vi "SFOAE-Init Level.vi"(0 "AO Runtime in":T2, 7 "DataProc In":T1, 11 "error in (no error)":errorcluster, 12 "Seq Step":i32, 13 "Lp (dB SPL)":cluster{"Min":dbl, "Max":dbl, "Step":dbl}) -> (3 "Lp":dbl, 4 "AO Runtime out":T2, 8 "Continue?":bool, 14 "DataProc Out":T1, 15 "error out":errorcluster)   [LabVIEW 2020]
uses:
  Typedefs/SFOAE-AO Runtime Data.ctl
  Typedefs/SFOAE-Data Processing.ctl
  epl-vi-lib/PXI DAQ VIs/DAQ Engine VIs/PXI Globals.vi
  epl-vi-lib/Utility VIs/Math VIs/dB to Linear (scalar).vi
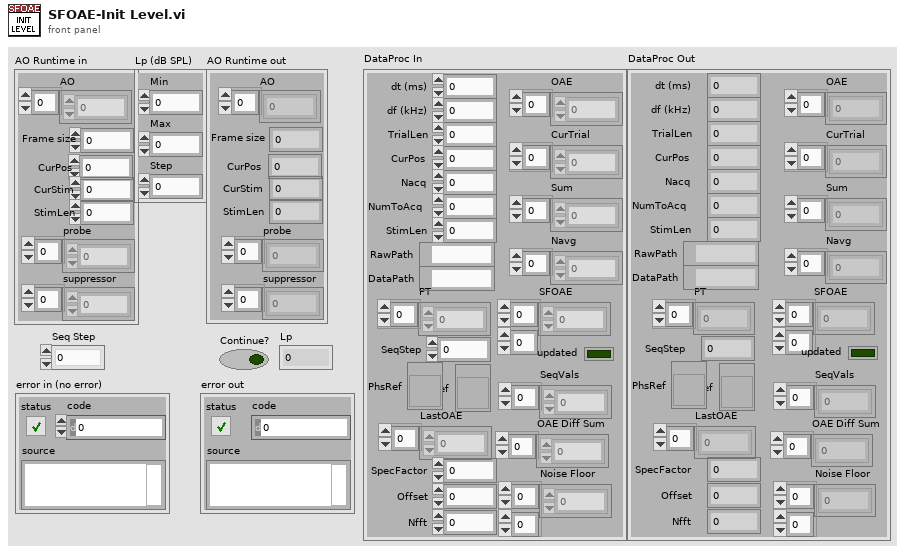
[diagram p1: front panel]
types:
  T1 = typedef "SFOAE-Data Processing.ctl" = cluster{"dt (ms)":dbl, "TrialLen":i32, "PT":cdb[], "CurPos":i32, "Sum":dbl[], "Navg":dbl[], "Nacq":i32, "RawPath":path, "DataPath":path, "NumToAcq":i32, "OAE":dbl[], "CurTrial":dbl[], "StimLen":i32, "SFOAE":cdb[][], "SeqStep":i32, "updated":bool, "SeqVals":dbl[], "df (kHz)":dbl, "MagRef":refnum<vi>, "LastOAE":dbl[], "OAE Diff Sum":dbl[], "Noise Floor":cdb[][], "SpecFactor":dbl, "Offset":i32, "Nfft":i32, "PhsRef":refnum<vi>}
  T2 = typedef "SFOAE-AO Runtime Data.ctl" = cluster{"AO":i32[], "Frame size":i32, "CurPos":i32, "probe":dbl[], "suppressor":dbl[], "CurStim":i32, "StimLen":i32}
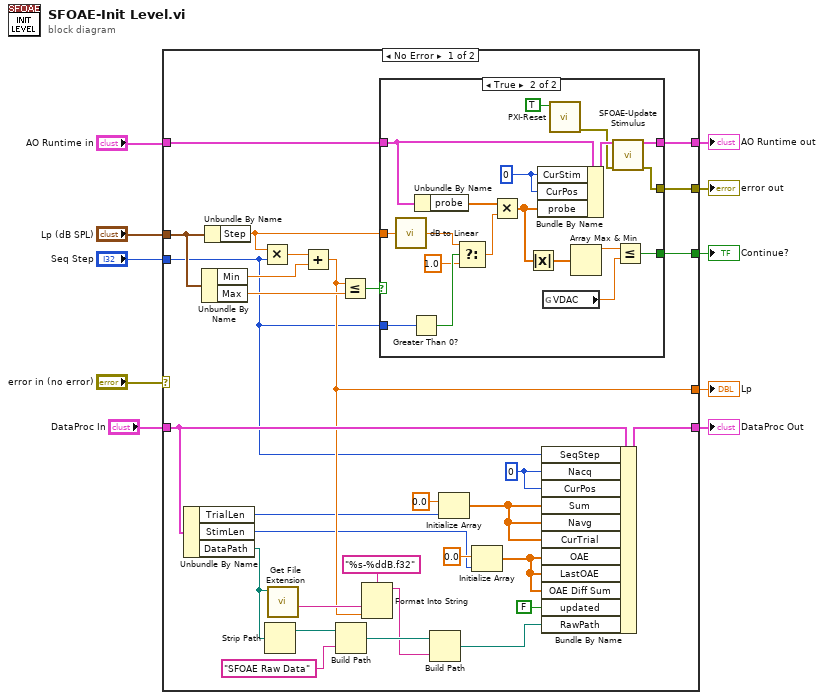
[diagram p0: block diagram]
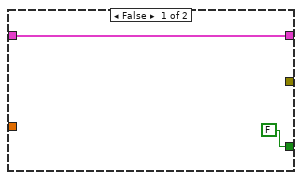
[diagram p2: hidden frame]
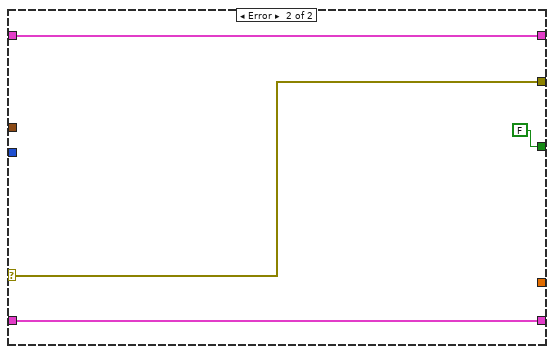
[diagram p3: hidden frame]
diagram:
  n1 = case shown="No Error" "error in (no error)" {
    selector: "error in (no error)" -> [_ w65]
    tunnel: "Lp (dB SPL)" -> [w34 _]
    tunnel: "AO Runtime in" -> [w38 w63]
    tunnel: [w37 w63] -> w8
    tunnel: [w31 w65] -> w9
    tunnel: [w32 FALSE ("Boolean")] -> w10
    tunnel: "Seq Step" -> [w11 _]
    tunnel: [w24 _] -> w3
    tunnel: [w29 w62] -> w2
    tunnel: "DataProc In" -> [w30 w62]
    frame No Error {
      w18 = 0 ("CurPos")
      n2 = Unbundle By Name(w30) -> ("TrialLen"=w15:i32, "StimLen"=w14:i32, "DataPath"=w27:path)
      n3 = Unbundle By Name(w34) -> ("Min"=w35:dbl, "Max"=w39:dbl)
      n4 = Unbundle By Name(w34) -> ("Step"=w33:dbl)
      n5 = Multiply(x=w33, y=w11) -> (x*y=w40:dbl)
      n6 = Strip Path(path=w27) -> (stripped path=w23:path)  [unwired: 1 out]
      n7 = call <vilib>:"Get File Extension.vi"("file"=w27) -> ("filename without extension"=w25:string)  [unwired: 6 in, 4 out]
      n8 = Add(x=w40, y=w35) -> (x+y=w24:dbl)
      n9 = Build Path(base path=w23, name or relative path="SFOAE Raw Data") -> (appended path=w22:path)
      n10 = Less Or Equal?(x=w24, y=w39) -> (x <= y?=w36:bool)
      n11 = Format Into String(format string="%s-%ddB.f32", w25, w24) -> (resulting string=w21:string)  [unwired: 2 in, 1 out]
      n12 = case shown="True" w36 {
        tunnel: w38 -> [w42 w61]
        tunnel: [w42 w53] -> w37
        tunnel: w33 -> [_ w59]
        tunnel: [FALSE w54] -> w32
        tunnel: [_ w51] -> w31
        tunnel: w11 -> [_ w50]
        frame False {
        }
        frame True {
          w43 = 0 ("CurPos")
          n13 = call-poly "dB to Linear.vi"("dB"=w59) -> ("linear"=w48:dbl)
          n14 = Greater Than 0?(x=w50) -> (x > 0?=w49:bool)
          n15 = Unbundle By Name(w61) -> ("probe"=w60:dbl[])
          n16 = Select(t=w48, s=w49, f=1.0) -> (s? t:f=w47:dbl)
          n17 = Multiply(x=w60, y=w47) -> (x*y=w55:dbl[])
          n18 = Absolute Value(x=w55) -> (abs(x)=w58:dbl[])
          n19 = Bundle By Name(cluster=w61, "CurStim"=w43, "CurPos"=w43, "probe"=w55) -> (w52:T2)
          n20 = global read "PXI Globals.vi" "VDAC"() -> (w56:dbl)
          n21 = call "PXI-Reset.vi"("Clear signal bank (F)"=TRUE) -> ("error out"=w45:errorcluster)  [unwired: 10 in]
          n22 = Array Max & Min(array=w58) -> (max value=w57:dbl)  [unwired: 3 out]
          n23 = call "SFOAE-Update Stimulus.vi"("AO Runtime in"=w52, "error in (no error)"=w45) -> ("AO Runtime out"=w53:T2, "error out"=w51:errorcluster)  [unwired: 12 in]
          n24 = Less Or Equal?(x=w57, y=w56) -> (x <= y?=w54:bool)
        }
      }
      n25 = Build Path(base path=w22, name or relative path=w21) -> (appended path=w20:path)
      n26 = Initialize Array(0.0 ("element"), w15) -> (w17:dbl[])
      n27 = Initialize Array(0.0 ("element"), w14) -> (w12:dbl[])
      n28 = Bundle By Name(cluster=w30, "SeqStep"=w11, "Nacq"=w18, "CurPos"=w18, "Sum"=w17, "Navg"=w17, "CurTrial"=w17, "OAE"=w12, "LastOAE"=w12, "OAE Diff Sum"=w12, "updated"=FALSE, "RawPath"=w20) -> (w29:T1)
    }
    frame Error {
    }
  }
  "Continue?" <- w10
  "error out" <- w9
  "AO Runtime out" <- w8
  "Lp" <- w3
  "DataProc Out" <- w2
